vi "drop db3 alarm.vi"(8 "error in (no error)":errorcluster) -> (0 "error out":errorcluster)   [LabVIEW 2016]
uses:
  <vilib>/addons/database/Connection.llb/DB Tools Open Connec (String).vi
  Access/Access Lib.lvlib
  <vilib>/addons/database/NI_Database_API.lvlib
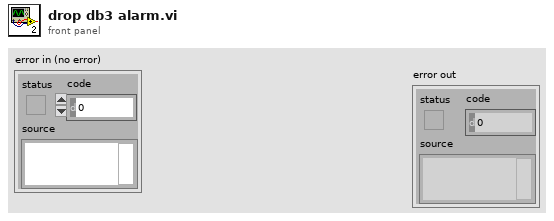
[diagram p1: front panel]
types:
  T1 = typedef "NI_Database_API.lvlib/Conn ObjectReference.ctl" = refnum<k1>
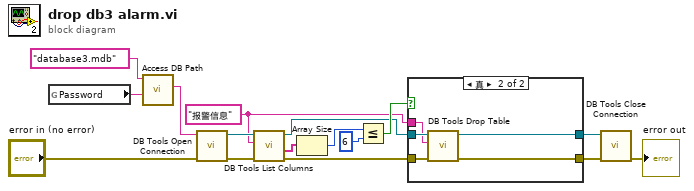
[diagram p0: block diagram]
diagram:
  w3 = "报警信息" ("table")
  n1 = global read "外部调用接口全局变量.vi" "Password"() -> (w1:string)
  n2 = call "Access DB Path.vi"("Password"=w1, "database"="database3.mdb") -> ("Connection information"=w16:string)  [unwired: 8 in, 1 out]
  n3 = call-poly <vilib>:"DB Tools Open Connection.vi"("error in (no error)"="error in (no error)", "connection information"=w16) -> ("error out"=w13:errorcluster, "connection reference"=w14:T1)  [unwired: 6 in]
  n4 = call <vilib>:"DB Tools List Columns.vi"("error in (no error)"=w13, "table"=w3, "connection reference"=w14) -> ("error out"=w6:errorcluster, "columns"=w11:string[], "connection reference out"=w7:T1)  [unwired: 1 in, 1 out]
  n5 = Array Size(array=w11) -> (size(s)=w10:i32)
  n6 = Less Or Equal?(x=w10, y=6) -> (x <= y?=w8:bool)
  n7 = case shown="真" w8 {
    tunnel: w7 -> [w18 w23]
    tunnel: w3 -> [_ w22]
    tunnel: w6 -> [w17 w21]
    tunnel: [w17 w20] -> w5
    tunnel: [w18 w19] -> w4
    frame False {
    }
    frame True {
      n8 = call <vilib>:"DB Tools Drop Table.vi"("error in (no error)"=w21, "table"=w22, "connection reference"=w23) -> ("error out"=w20:errorcluster, "connection reference out"=w19:T1)  [unwired: 5 in]
    }
  }
  n9 = call <vilib>:"DB Tools Close Connection.vi"("error in (no error)"=w5, "connection reference"=w4) -> ("error out"=→"error out":errorcluster)  [unwired: 5 in]
